vi "Position_Debug_r1.vi"() -> ()   [LabVIEW 2015]
panel:
  in  "goal x":dbl=0.25 format="%#_13g"
  in  "start x":dbl=0.25 format="%#_13g"
  in  "goal y 2":dbl=0.25 format="%#_13g"
  in  "start y":dbl=0.25 format="%#_13g"
  out "Wheel  PID SetPoint output Array":dbl[](array[numeric])
  out "Wheel  PID SetPoint input Array":dbl[](array[numeric])
  out "omega and angular velocity calc input array":dbl[](array[numeric])
  out "omega and angular velocity calc output array":dbl[](array[numeric])
  in  "Phi Current":dbl format="%#_13g"
  in  "phi old":dbl
  in  "y traveled old":dbl
  in  "x traveled old":dbl
  out "y traveled new":dbl
  out "y position":dbl
  out "x traveled new":dbl
  out "x position":dbl
  out "phi new":dbl
  out "x & y position input array":dbl[](array[numeric])
  out "x & y position output array":dbl[](array[numeric])
  out "encoder step sub vi output":dbl[](array[numeric])
  out "encoder sub vi input array":dbl[](array[numeric])
  out "Distance Step":dbl
  out "Avg L Step":dbl
  out "Avg L Dist New":dbl
  out "Avg R Step":dbl
  out "Avg R Dist New":dbl
  in  "Avg L Dist Old":dbl
  in  "Avg R Dist Old":dbl
  out "track width(ft)":dbl=4.0
  out "Tick Count(mSec) 2":u32 caption="Tick Count(mSec)"
  out "Left Setpoint":dbl
  out "Right Setpoint":dbl
  out "robot desired velocity y component\n u2 (ft/s)":dbl
  out "robot desired velocity x component\n u1 (ft/s)":dbl
  out "Desired Velocity":dbl
  out "Reset X Y":dbl
  out "Scale":dbl=1.0
  out "y position":dbl
  out "x traveled 2":dbl
  out "Omega":dbl format="%.2f"
  out "Phi desired":dbl
  out "v right wheel":dbl
  out "v left wheel":dbl
  out "max v":dbl
  out "loc_x":dbl
  out "loc_flag":bool
  out "x delta":dbl
  out "x position camera":dbl
  in  "Encoder Reset":bool
  out "RM Distance (ft)":dbl
  out "RR Distance (ft)":dbl
  out "LF Distance (ft)":dbl
  out "LM Distance (ft)":dbl
  out "RF Distance (ft)":dbl
  out "LR Distance (ft)":dbl
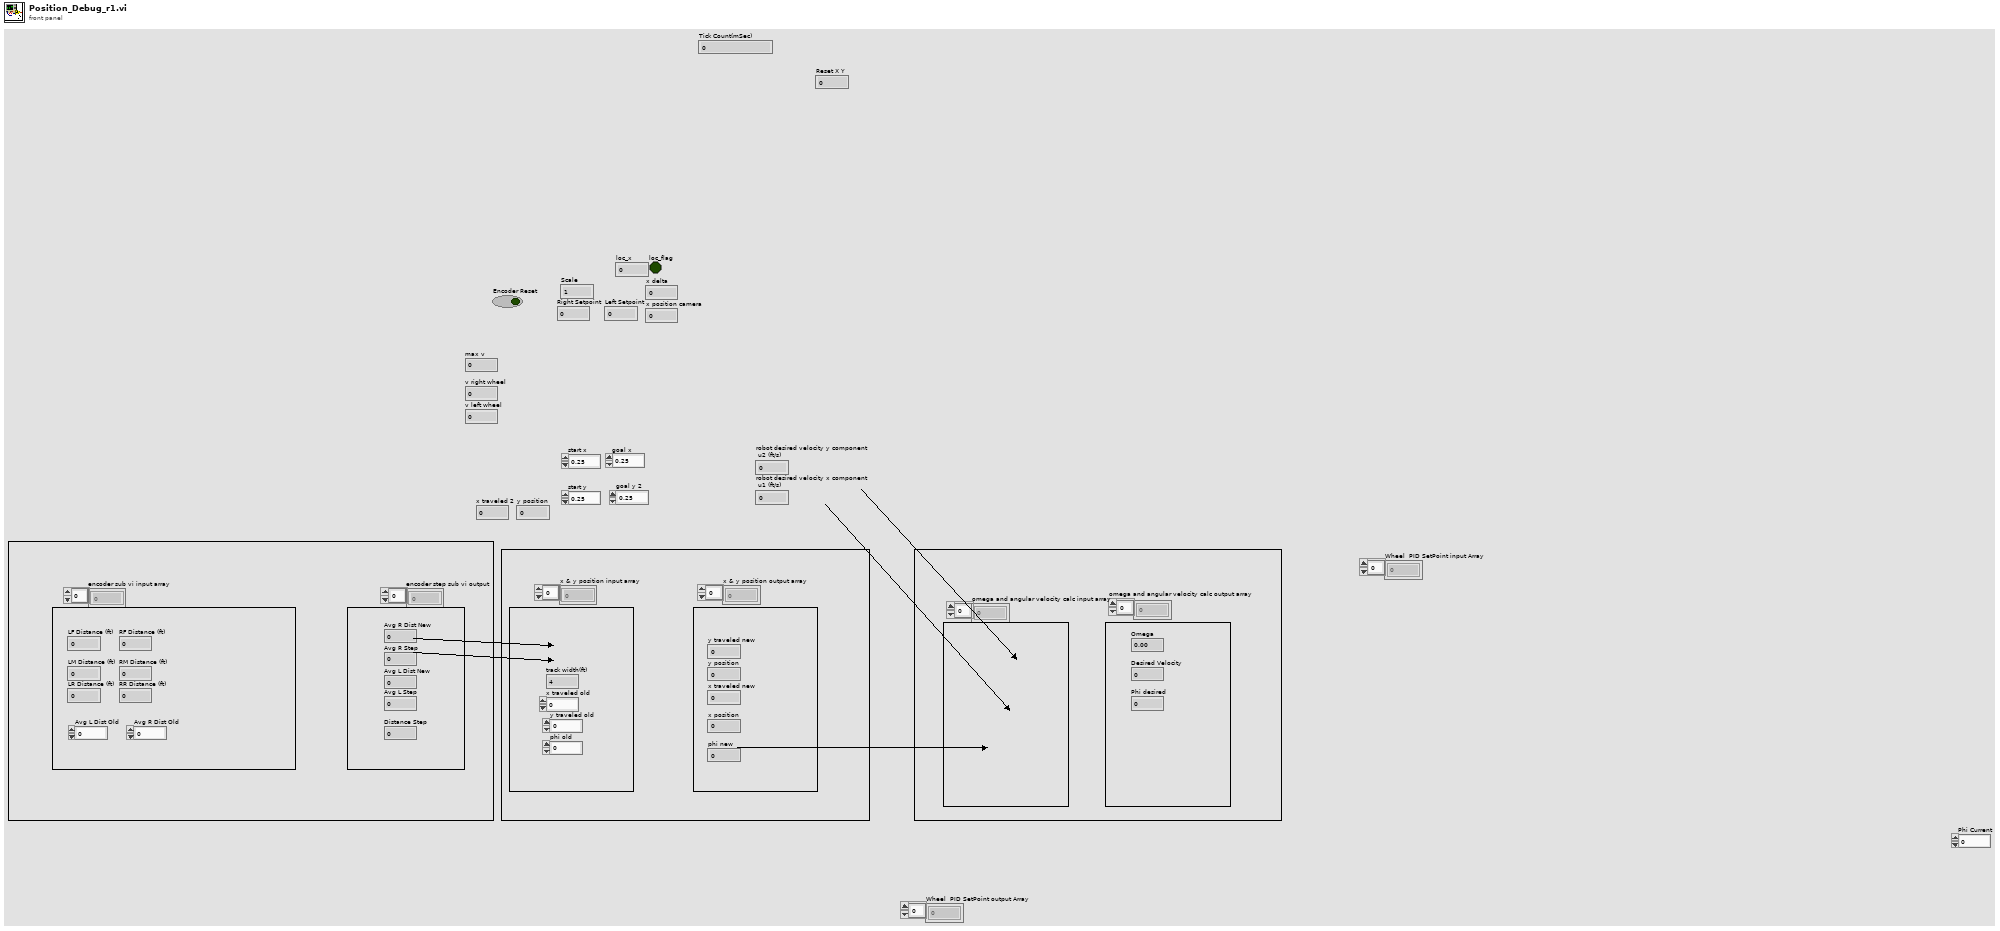
[diagram p1: front panel]
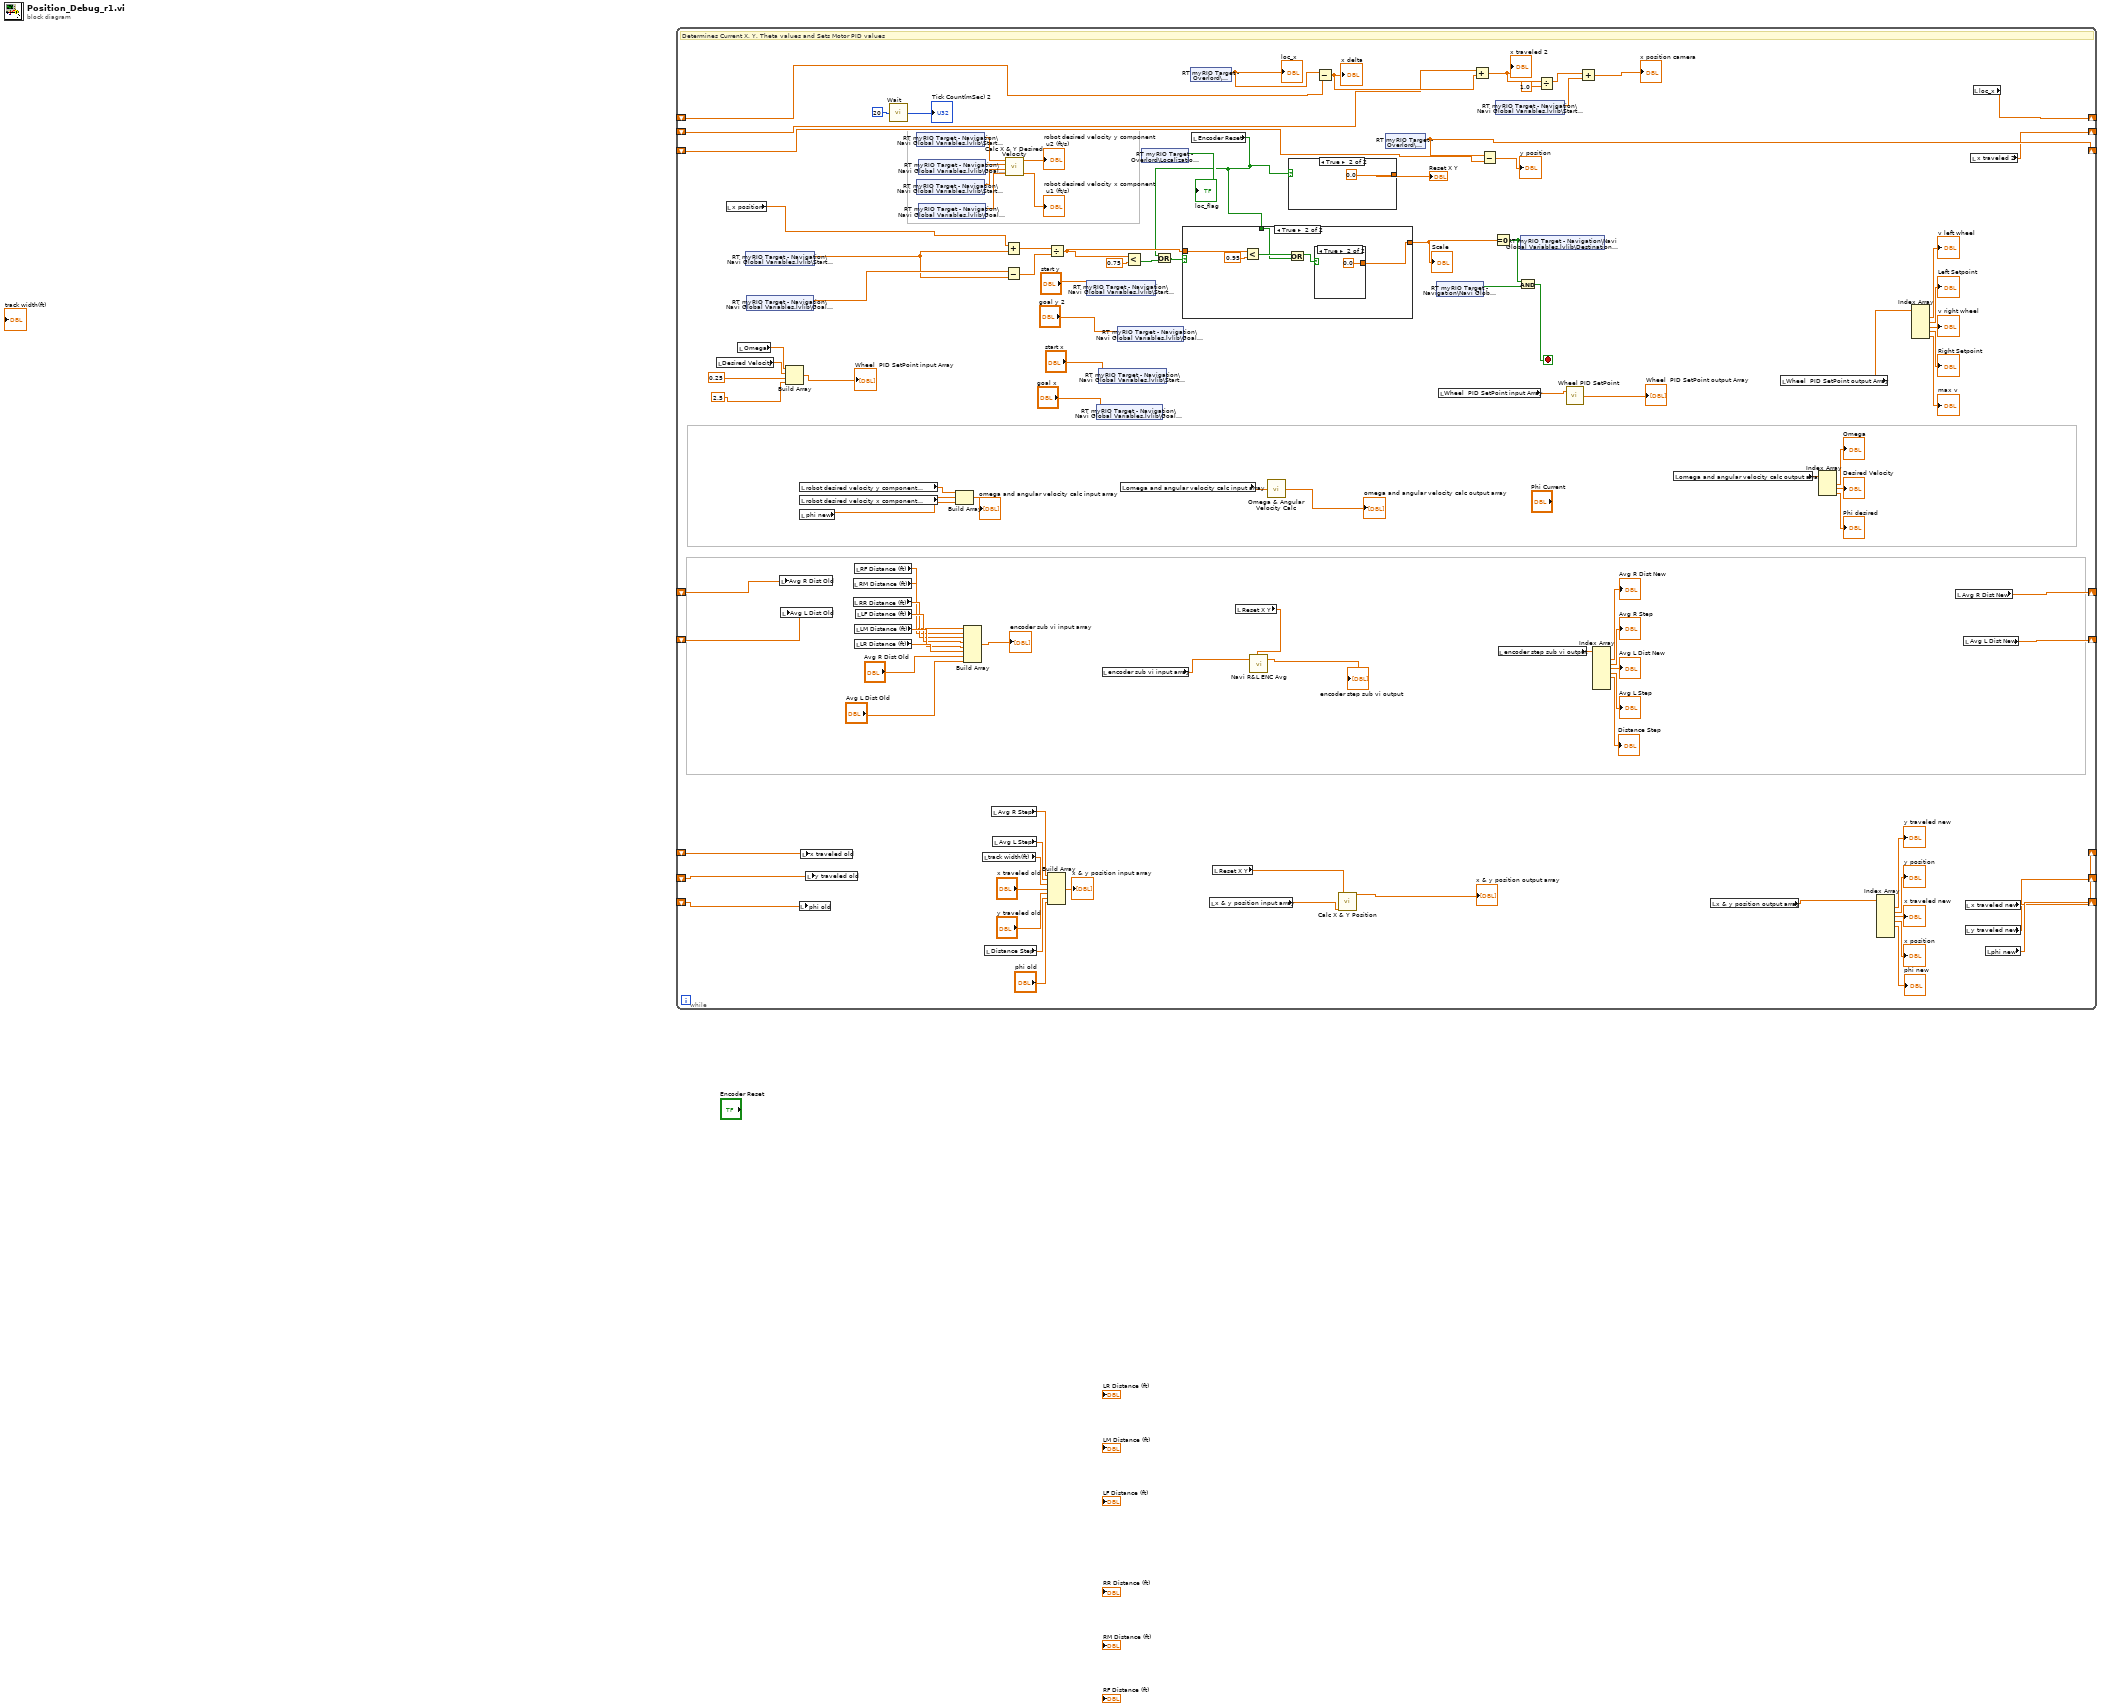
[diagram p0: block diagram]
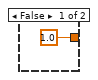
[diagram p2: hidden frame]
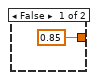
[diagram p3: hidden frame]
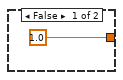
[diagram p4: hidden frame]
diagram:
  n1 = while {
    shift-right: [w81] -> _
    shift-left: _ -> [w83]
    shift-right: [w89] -> _
    shift-left: _ -> [w90]
    shift-right: [w78] -> _
    shift-left: _ -> [w79]
    shift-right: [w40] -> _
    shift-left: _ -> [w62]
    shift-right: [w41] -> _
    shift-left: _ -> [w63]
    shift-right: [w37] -> _
    shift-left: _ -> [w31]
    shift-right: [w38] -> _
    shift-left: _ -> [w32]
    shift-right: [w39] -> _
    shift-left: _ -> [w30]
    stop <- w106 stop-if-true
    # "Determines Current X, Y, Theta values and Sets Motor PID values"
    n2 = local read "Desired Velocity"() -> (w17:dbl)
    n3 = local read "x position"() -> (w87:dbl)
    n4 = local read "Omega"() -> (w16:dbl)
    n5 = shared-variable "RT myRIO Target - Navigation\\Navi Global Variables.lvlib\\Start Position X"() -> (w82:dbl)  [unwired: 1 in, 1 out]
    n6 = shared-variable "RT myRIO Target - Navigation\\Navi Global Variables.lvlib\\Goal Position X"() -> (w95:dbl)  [unwired: 1 in, 1 out]
    n7 = local write "Avg R Dist Old"(w63) -> ()
    n8 = local write "Avg L Dist Old"(w62) -> ()
    n9 = Build Array(w16, w17, 0.25 ("element"), 2.5 ("element")) -> (→"Wheel  PID SetPoint input Array":dbl[])
    n10 = local write "phi old"(w30) -> ()
    n11 = local read "robot desired velocity y component\n u2 (ft/s)"() -> (w23:dbl)
    n12 = local read "robot desired velocity x component\n u1 (ft/s)"() -> (w25:dbl)
    n13 = local read "phi new"() -> (w24:dbl)
    n14 = local write "x traveled old"(w32) -> ()
    n15 = local write "y traveled old"(w31) -> ()
    n16 = local read "RM Distance (ft)"() -> (w54:dbl)
    n17 = local read "RR Distance (ft)"() -> (w55:dbl)
    n18 = local read "RF Distance (ft)"() -> (w53:dbl)
    n19 = local read "LM Distance (ft)"() -> (w57:dbl)
    n20 = local read "LR Distance (ft)"() -> (w58:dbl)
    n21 = local read "LF Distance (ft)"() -> (w56:dbl)
    n22 = call "Wait"("Count(mSec)"=u32 20) -> ("Tick Count(mSec)"=→"Tick Count(mSec) 2":u32)
    n23 = shared-variable "RT myRIO Target - Navigation\\Navi Global Variables.lvlib\\Start Position Y"() -> (w105:dbl)  [unwired: 1 in, 1 out]
    n24 = shared-variable "RT myRIO Target - Navigation\\Navi Global Variables.lvlib\\Start Position X"() -> (w103:dbl)  [unwired: 1 in, 1 out]
    n25 = shared-variable "RT myRIO Target - Navigation\\Navi Global Variables.lvlib\\Goal Position Y"() -> (w104:dbl)  [unwired: 1 in, 1 out]
    n26 = shared-variable "RT myRIO Target - Navigation\\Navi Global Variables.lvlib\\Goal Position X"() -> (w102:dbl)  [unwired: 1 in, 1 out]
    n27 = Build Array(w23, w25, w24) -> (→"omega and angular velocity calc input array":dbl[])
    n28 = Build Array(w53, w54, w55, w56, w57, w58, "Avg R Dist Old", "Avg L Dist Old") -> (→"encoder sub vi input array":dbl[])
    n29 = local read "track width(ft)"() -> (w50:dbl)
    n30 = local read "Distance Step"() -> (w34:dbl)
    n31 = local read "Avg R Step"() -> (w52:dbl)
    n32 = local read "Avg L Step"() -> (w51:dbl)
    n33 = Add(x=w87, y=w82) -> (x+y=w98:dbl)
    n34 = Subtract(x=w95, y=w82) -> (x-y=w96:dbl)
    n35 = call "Calc X & Y Desired Velocity.vi"("x goal"=w102, "x start"=w103, "Y Goal"=w104, "Y Position"=w105) -> ("robot desired velocity x component\n u1 (ft/s)"=→"robot desired velocity x component\n u1 (ft/s)":dbl, "robot desired velocity y component\n u2 (ft/s)"=→"robot desired velocity y component\n u2 (ft/s)":dbl)  [unwired: 6 in]
    n36 = Build Array(w52, w51, w50, "x traveled old", "y traveled old", w34, "phi old") -> (→"x & y position input array":dbl[])
    n37 = Divide(x=w98, y=w96) -> (x/y=w97:dbl)
    n38 = shared-variable "RT myRIO Target - Navigation\\Navi Global Variables.lvlib\\Start Position Y"("start y") -> ()  [unwired: 1 in, 1 out]
    n39 = shared-variable "RT myRIO Target - Navigation\\Navi Global Variables.lvlib\\Goal Position X"("goal x") -> ()  [unwired: 1 in, 1 out]
    n40 = shared-variable "RT myRIO Target - Navigation\\Navi Global Variables.lvlib\\Start Position X"("start x") -> ()  [unwired: 1 in, 1 out]
    n41 = local read "encoder sub vi input array"() -> (w71:dbl[])
    n42 = shared-variable "RT myRIO Target - Navigation\\Navi Global Variables.lvlib\\Goal Position Y"("goal y 2") -> ()  [unwired: 1 in, 1 out]
    n43 = local read "omega and angular velocity calc input array"() -> (w26:dbl[])
    n44 = Less?(x=w97, y=0.75) -> (x < y?=w86:bool)
    n45 = shared-variable "RT myRIO Target - Overlord\\Localization_Variables_r0.lvlib\\loc_flag"() -> (→"loc_flag":bool)  [unwired: 1 in, 1 out]
    n46 = shared-variable "RT myRIO Target - Overlord\\Localization_Variables_r0.lvlib\\loc_x"() -> (w91:dbl)  [unwired: 1 in, 1 out]
    "loc_x" <- w91
    n47 = local read "Encoder Reset"() -> (w84:bool)
    n48 = Or(x=w84, y=w86) -> (x .or. y?=w92:bool)
    n49 = case shown="True" w92 {
      tunnel: w97 -> [_ w117]
      tunnel: [1.0 w114] -> w93
      tunnel: w84 -> [_ w112]
      frame False {
      }
      frame True {
        n50 = Less?(x=w117, y=0.95) -> (x < y?=w115:bool)
        n51 = Or(x=w115, y=w112) -> (x .or. y?=w113:bool)
        n52 = case shown="True" w113 {
          tunnel: [0.85 0.0] -> w114
          frame False {
          }
          frame True {
          }
        }
      }
    }
    "Scale" <- w93
    n53 = local read "x & y position input array"() -> (w29:dbl[])
    n54 = local read "Reset X Y"() -> (w28:dbl)
    n55 = local read "Reset X Y"() -> (w72:dbl)
    n56 = call "Navi R&L ENC Avg.vi"("encoder step sub vi input"=w71, "Reset X Y"=w72) -> ("encoder step sub vi output"=→"encoder step sub vi output":dbl[])  [unwired: 17 in]
    n57 = call "Omega & Angular Velocity Calc.vi"("omega and angular velocity calc input array"=w26) -> ("omega and angular velocity calc output array"=→"omega and angular velocity calc output array":dbl[])  [unwired: 4 in]
    n58 = case shown="True" w84 {
      tunnel: [1.0 0.0] -> w99
      frame False {
      }
      frame True {
      }
    }
    "Reset X Y" <- w99
    n59 = Subtract(x=w91, y=w83) -> (x-y=w80:dbl)
    "x delta" <- w80
    n60 = call "Calc X & Y Position.vi"("x & y position input array"=w29, "Reset X Y"=w28) -> ("y & x traveled output array"=→"x & y position output array":dbl[])  [unwired: 16 in, 1 out]
    n61 = shared-variable "RT myRIO Target - Overlord\\Localization_Variables_r0.lvlib\\loc_y"() -> (w89:dbl)  [unwired: 1 in, 1 out]
    n62 = shared-variable "RT myRIO Target - Navigation\\Navi Global Variables.lvlib\\All Stop"() -> (w108:bool)  [unwired: 1 in, 1 out]
    n63 = local read "Wheel  PID SetPoint input Array"() -> (w12:dbl[])
    n64 = Add(x=w79, y=w80) -> (x+y=w76:dbl)
    "x traveled 2" <- w76
    n65 = Subtract(x=w89, y=w90) -> (x-y=→"y position":dbl)
    n66 = Equal To 0?(x=w93) -> (x = 0?=w107:bool)
    n67 = shared-variable "RT myRIO Target - Navigation\\Navi Global Variables.lvlib\\Start Position X"() -> (w77:dbl)  [unwired: 1 in, 1 out]
    n68 = local read "encoder step sub vi output"() -> (w66:dbl[])
    n69 = And(x=w107, y=w108) -> (x .and. y?=w106:bool)
    n70 = shared-variable "RT myRIO Target - Navigation\\Navi Global Variables.lvlib\\Destination Reached"(w107) -> ()  [unwired: 1 in, 1 out]
    n71 = Divide(x=w76, y=1.0) -> (x/y=w74:dbl)
    n72 = call "Wheel PID SetPoint.vi"("Wheel  PID SetPoint Input Array"=w12) -> ("Wheel  PID SetPoint output Array"=→"Wheel  PID SetPoint output Array":dbl[])  [unwired: 1 in]
    n73 = Add(x=w74, y=w77) -> (x+y=→"x position camera":dbl)
    n74 = Index Array(array=w66) -> (element #1=→"Avg R Dist New":dbl, element #2=→"Avg R Step":dbl, element #3=→"Avg L Dist New":dbl, element #4=→"Avg L Step":dbl, element #5=→"Distance Step":dbl)  [unwired: 7 in, 2 out]
    n75 = local read "omega and angular velocity calc output array"() -> (w21:dbl[])
    n76 = local read "x & y position output array"() -> (w45:dbl[])
    n77 = local read "Wheel  PID SetPoint output Array"() -> (w10:dbl[])
    n78 = Index Array(array=w21) -> (element #1=→"Omega":dbl, element #2=→"Desired Velocity":dbl, element #3=→"Phi desired":dbl)  [unwired: 3 in]
    n79 = Index Array(array=w45) -> (element #1=→"y traveled new":dbl, element #2=→"y position":dbl, element #3=→"x traveled new":dbl, element #4=→"x position":dbl, element #5=→"phi new":dbl)  [unwired: 7 in, 2 out]
    n80 = Index Array(array=w10) -> (element #1=→"v left wheel":dbl, element #2=→"Left Setpoint":dbl, element #3=→"v right wheel":dbl, element #4=→"Right Setpoint":dbl, element #5=→"max v":dbl)  [unwired: 5 in]
    n81 = local read "Avg R Dist New"() -> (w41:dbl)
    n82 = local read "Avg L Dist New"() -> (w40:dbl)
    n83 = local read "x traveled new"() -> (w38:dbl)
    n84 = local read "y traveled new"() -> (w37:dbl)
    n85 = local read "x traveled 2"() -> (w78:dbl)
    n86 = local read "loc_x"() -> (w81:dbl)
    n87 = local read "phi new"() -> (w39:dbl)
  }
